vi "Convert messages to String.vi"(9 "Command":T1=enum."MCU Reset", 10 "TestName":string, 11 "Communication":T2(array[cluster])) -> (3 "String":string)   [LabVIEW 2025]
uses:
  Communication Handle/API/Commands.ctl
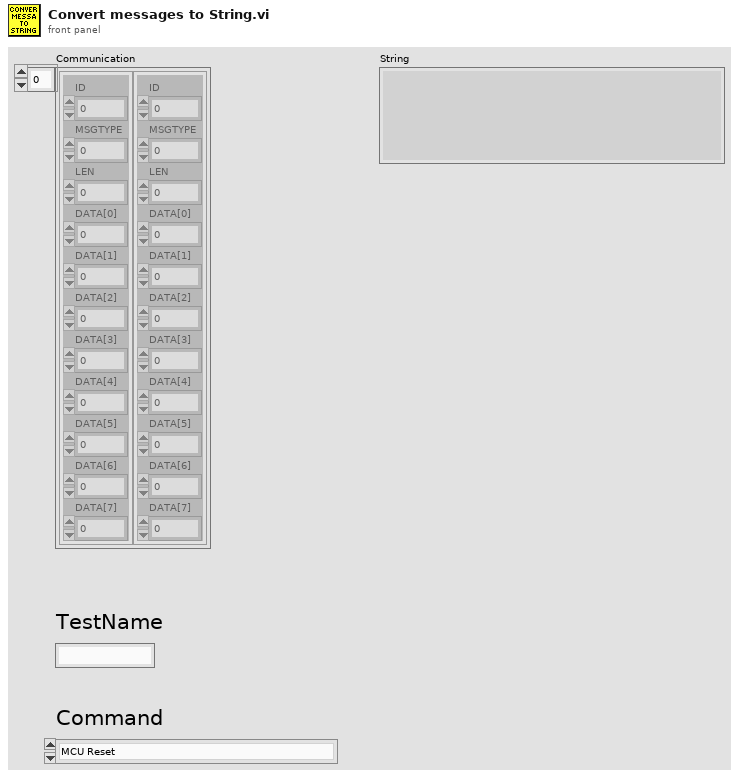
[diagram p1: front panel]
types:
  T1 = typedef "Commands.ctl" = enum16{"Nexteer connect", "Write Polarity", "Write BEMF", "Write Torque Scale Sensors T1", "Write Torque Scale Sensors T2", "Trim HW Torque Sensors T1", "Trim HW Torque Sensors T2", "Read HW Torque Trim Performed Sensors T1", "Read HW Torque Trim Performed Sensors T2", "Write EOL Offset values to defaults", "Write EOL Gain values to defaults", "Write Serial Number", "Write Hardware Part Number", "Write EPS Serial Number", "Read MEC Counter", "MCU Reset", "Read System State", "Read First Motor Position", "Manufacturing Diagnostic Defeat", "Perform Current Offset ", "Current Offset Status", "Enable Engine Run", "Perform Current Gain ", "Current Gain Status", "Disable Torque Ramp Down ", "Disable Engine Run", "Set Vehicle Speed Override", "Read Offset Values Using FD F5", "Read Gain Values Using FD F4", "Clear Nexteer NTCs", "Read Second Motor Position", "Read ECU Software ID", "Read Internal Software Version", "Read Bootloader ID", "Read Bootloader Software Version", "Read Calibration Release 0", "Read Calibration Release 1", "Read Calibration Release 2", "Read Temperature  ", "Battery Voltage  ", "Read Motor Angle 0", "Read Motor Angle 1 ", "Set Motor Torque Command ", "Read Motor Current   ", "Stop Motor Torque Command", "Read NTCs", "Read Serial Number", "Read HW Part Number", "Read Polarity", "Set NVM Access Defeat", "Read Software Release", "Read Software Build Date", "Write Single Inverter Hardware value", "Write Dual Inverter Hardware value", "Read Single Inverter HW Value", "Read Dual Inverter HW Value", "Write MEC Counter FE", "Write MEC Counter FF", "Read BEMF", "Read Torque 1 FDB6", "Read Torque 2 FDB7", "Read Torque Trim 1 FDB4", "Read Torque Trim 2 FDB5", "Write Torque Trim 1 FDB4", "Write Torque Trim 2 FDB5", "XCP connect", "Read HW Torque T1", "Read HW Torque T2", "Read Motor Speed "}
  T2 = cluster{"ID":u32, "MSGTYPE":u8, "LEN":u8, "DATA[0]":u8, "DATA[1]":u8, "DATA[2]":u8, "DATA[3]":u8, "DATA[4]":u8, "DATA[5]":u8, "DATA[6]":u8, "DATA[7]":u8}[]
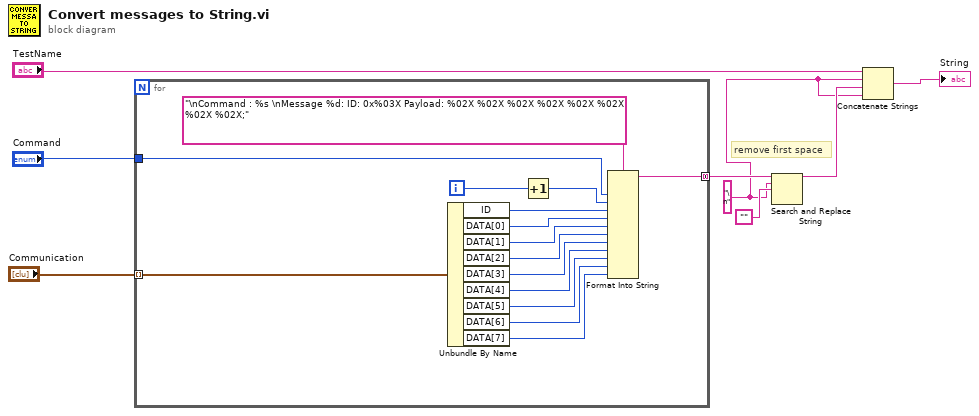
[diagram p0: block diagram]
diagram:
  w1 = "\n" ("search string")
  # "remove first space"
  n1 = for {
    tunnel: "Communication" -> [w23] mode=indexing
    tunnel: [w22] -> w7 mode=concatenating
    tunnel: "Command" -> [w9]
    i -> [w20]
    n2 = Unbundle By Name(w23) -> ("ID"=w11:u32, "DATA[0]"=w19:u8, "DATA[1]"=w18:u8, "DATA[2]"=w17:u8, "DATA[3]"=w16:u8, "DATA[4]"=w15:u8, "DATA[5]"=w14:u8, "DATA[6]"=w13:u8, "DATA[7]"=w12:u8)
    n3 = Increment(x=w20) -> (x+1=w10:i32)
    n4 = Format Into String(format string="\nCommand : %s \nMessage %d: ID: 0x%03X Payload: %02X %02X %02X %02X %02X %02X %02X %02X;", w9, w10, w11, w19, w18, w17, w16, w15, w14, w13, w12) -> (resulting string=w22:string)  [unwired: 2 in, 1 out]
  }
  n5 = Search and Replace String(input string=w7, search string=w1, replace string="") -> (result string=w4:string)  [unwired: 5 in, 3 out]
  n6 = Concatenate Strings("TestName", w1, w4, w1) -> (→"String":string)
